vi "AO Pattern Generation.vi"(8 "error in":errorcluster, 10 "Timing":T2={"samples per channel"=1000, "sample mode"=10178, "Sampling Rate"=1000.0} {"sample mode" items=["Finite Samples"=10178, "Continuous Samples"=10123, "Hardware Timed Single Point"=12522]}, 11 "Config":T1[](array[typedef])) -> (0 "error out":errorcluster, 3 "Config":T1[](array[typedef]))   [LabVIEW 2024]
doc: "All Rights Reserved © 2017 SyncSols"
uses:
  Controls/AO Channel Configuration Cluster.ctl
  Controls/AO Timing Cluster.ctl
  <vilib>/measure/NI_MABase.lvlib
  <vilib>/Analysis/NI_AALBase.lvlib
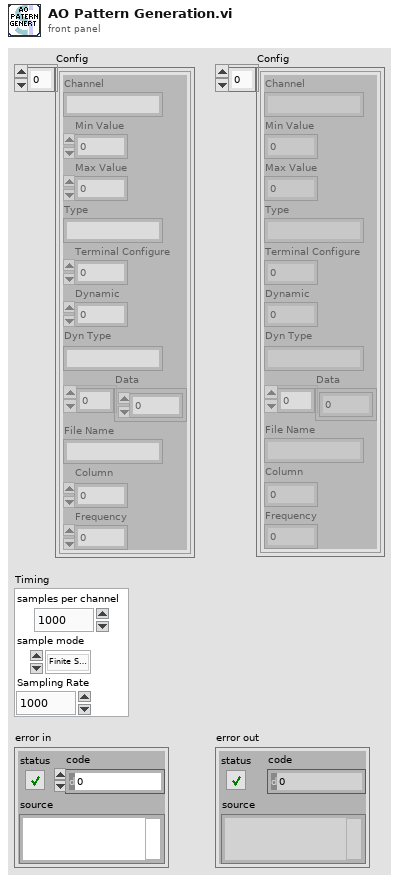
[diagram p1: front panel]
types:
  T1 = typedef "AO Channel Configuration Cluster.ctl" = cluster{"Channel":string, "Min Value":dbl, "Max Value":dbl, "Type":string, "Terminal Configure":u16, "Dynamic":u8, "Dyn Type":string, "Data":dbl[], "File Name":string, "Column":i32, "Frequency":dbl}
  T2 = typedef "AO Timing Cluster.ctl" = cluster{"samples per channel":i32, "sample mode":i32, "Sampling Rate":dbl}
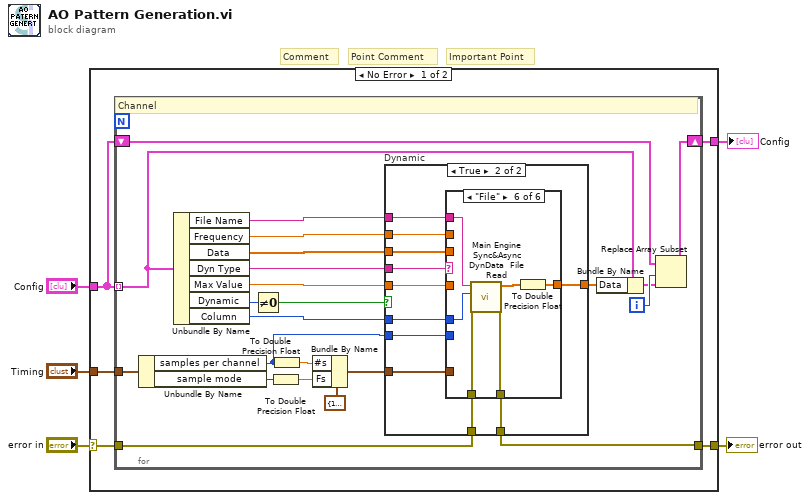
[diagram p0: block diagram]
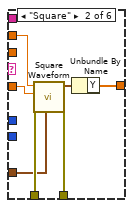
[diagram p4: hidden frame]
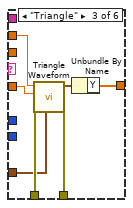
[diagram p5: hidden frame]
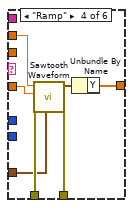
[diagram p6: hidden frame]
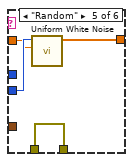
[diagram p7: hidden frame]
diagram:
  # "Important Point"
  # "Point Comment"
  # "Comment"
  n1 = case shown="No Error" "error in" {
    selector: "error in" -> [w10 w81]
    tunnel: [w9 w81] -> w5
    tunnel: "Config" -> [w7 w80]
    tunnel: "Timing" -> [w8 _]
    tunnel: [w6 w80] -> w1
    frame No Error {
      n2 = for {
        tunnel: w7 -> [w19] mode=indexing
        tunnel: w10 -> [w29]
        tunnel: [w28] -> w9
        tunnel: w8 -> [w27]
        shift-right: [w15] -> w6
        shift-left: w7 -> [w17]
        i -> [w20]
        # "Channel"
        n3 = Unbundle By Name(w27) -> ("samples per channel"=w14:i32, "sample mode"=w25:i32)
        n4 = Unbundle By Name(w19) -> ("File Name"=w12:string, "Frequency"=w13:dbl, "Data"=w21:dbl[], "Dyn Type"=w33:string, "Max Value"=w30:dbl, "Dynamic"=w32:u8, "Column"=w11:i32)
        n5 = Not Equal To 0?(x=w32) -> (x != 0?=w31:bool)
        n6 = To Double Precision Float(number=w25) -> (double precision float=w24:dbl)
        n7 = To Double Precision Float(number=w14) -> (double precision float=w23:dbl)
        n8 = Bundle By Name(cluster=cluster{"Fs":dbl, "#s":dbl} {"Fs"=1000.0, "#s"=1000.0} ("sampling info"), "#s"=w23, "Fs"=w24) -> (w22:cluster{"Fs":dbl, "#s":dbl})
        n9 = case "Dynamic" shown="True" w31 {
          tunnel: w33 -> [_ w46]
          tunnel: w30 -> [_ w38]
          tunnel: w29 -> [w34 w45]
          tunnel: [w34 w44] -> w28
          tunnel: w13 -> [_ w43]
          tunnel: w22 -> [_ w42]
          tunnel: w21 -> [w35 w40]
          tunnel: [w35 w41] -> w18
          tunnel: w14 -> [_ w39]
          tunnel: w12 -> [_ w37]
          tunnel: w11 -> [_ w36]
          frame False {
          }
          frame True {
            n10 = case shown="\"File\"" w46 {
              tunnel: w45 -> [w47 w55 w62 w69 w71 w77]
              tunnel: [w47 w54 w61 w68 w71 w76] -> w44
              tunnel: w43 -> [_ w53 w60 w67 _ _]
              tunnel: w38 -> [_ w52 w59 w66 w72 _]
              tunnel: w42 -> [_ w51 w58 w65 _ _]
              tunnel: [w48 w49 w56 w63 w70 w74] -> w41
              tunnel: w40 -> [w48 _ _ _ _ _]
              tunnel: w39 -> [_ _ _ _ w73 _]
              tunnel: w37 -> [_ _ _ _ _ w79]
              tunnel: w36 -> [_ _ _ _ _ w78]
              frame Default {
              }
              frame "Square" {
                n11 = call <vilib>:"Square Waveform.vi"("sampling info"=w51, "error in (no error)"=w55, "amplitude"=w52, "frequency"=w53) -> ("error out"=w54:errorcluster, "signal out"=w50:waveform(dbl))  [unwired: 6 in]
                n12 = Unbundle By Name(w50) -> ("Y"=w49:dbl[])
              }
              frame "Triangle" {
                n13 = call <vilib>:"Triangle Waveform.vi"("sampling info"=w58, "error in (no error)"=w62, "amplitude"=w59, "frequency"=w60) -> ("error out"=w61:errorcluster, "signal out"=w57:waveform(dbl))  [unwired: 6 in]
                n14 = Unbundle By Name(w57) -> ("Y"=w56:dbl[])
              }
              frame "Ramp" {
                n15 = call <vilib>:"Sawtooth Waveform.vi"("sampling info"=w65, "error in (no error)"=w69, "amplitude"=w66, "frequency"=w67) -> ("error out"=w68:errorcluster, "signal out"=w64:waveform(dbl))  [unwired: 6 in]
                n16 = Unbundle By Name(w64) -> ("Y"=w63:dbl[])
              }
              frame "Random" {
                n17 = call <vilib>:"Uniform White Noise.vi"("amplitude"=w72, "samples"=w73) -> ("uniform white noise"=w70:dbl[])  [unwired: 8 in, 1 out]
              }
              frame "File" {
                n18 = call "Main Engine Sync&Async DynData  File Read.vi"("error in"=w77, "Column"=w78, "File Name"=w79) -> ("error out"=w76:errorcluster, "File DynData"=w75:sgl[])  [unwired: 7 in]
                n19 = To Double Precision Float(number=w75) -> (double precision float=w74:dbl[])
              }
            }
          }
        }
        n20 = Bundle By Name(cluster=w19, "Data"=w18) -> (w16:T1)
        n21 = Replace Array Subset(array=w17, new element=w16, index=w20) -> (w15:T1[])
      }
    }
    frame Error {
    }
  }
  "error out" <- w5
  "Config" <- w1
